vi "Real-Time Main-Final_Local_Digital_V2.vi"() -> ()   [LabVIEW 2024]
uses:
  <instrlib>/niScope/Controls/niScope trigger source digital.ctl
  <vilib>/Platform/TimedLoop/XDataNode/timing_clust.ctl
  <vilib>/Platform/TimedLoop/XDataNode/nitl_modes.ctl
  <vilib>/Platform/TimedLoop/XDataNode/wakeup.ctl
  <instrlib>/niScope/Configure/Trigger/niScope Configure Trigger Digital.vi
  <instrlib>/niScope/Acquire/Fetch/niScope Fetch WDT.vi
  <vilib>/Waveform/WDTOps.llb/WDT Get Waveform Time Array DBL.vi
  <vilib>/platform/TimedLoop/XDataNode/XDataNode.xnode
  <vilib>/Platform/TimedLoop/XDataNode/XDNodeRunTimeDep.lvlib
panel:
  in  "channels":string="0"
  in  "FileName":string
  out "# of Chunks Fetched":i32
  out "# of Points Fetched":i32
  in  "stop":bool
  in  "Fetch:Fetch Relative To":i32(ring)=482 items=["Start"=482, "Trigger"=483, "Pretrigger"=477, "Now"=481, "Read Pointer"=388]
  out "wfm":waveform(dbl)(graph)
  out "Time_shift":dbl
  in  "Resource Name":refnum<k15>="Dev1" caption="Resource Name(s)"
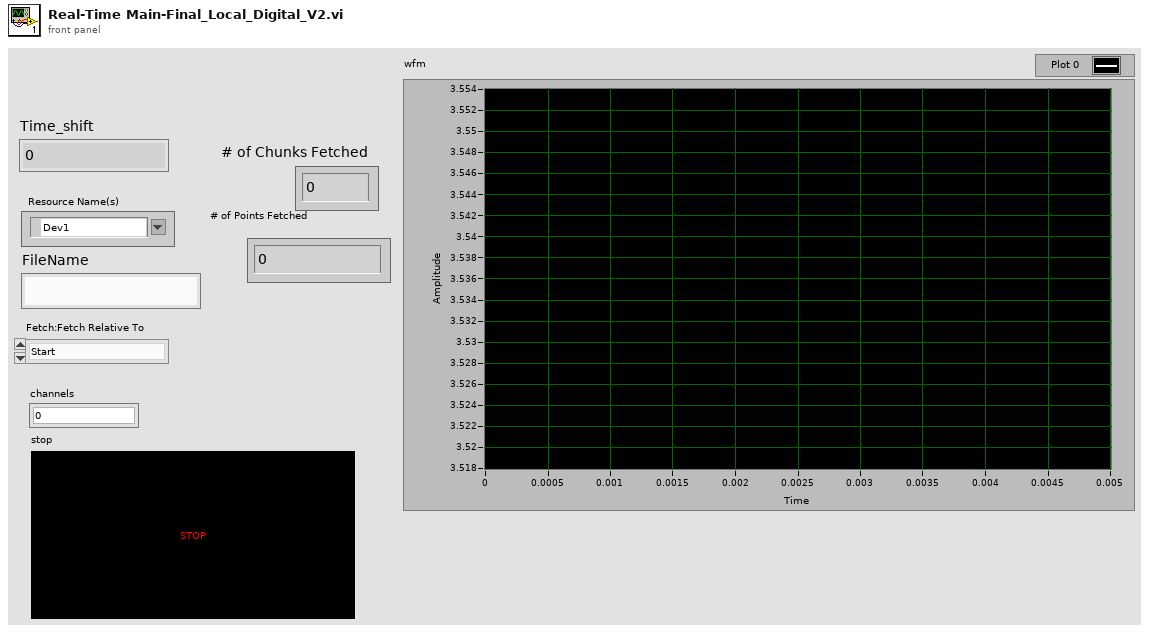
[diagram p1: front panel]
types:
  T1 = typedef "niScope trigger source digital.ctl" = string
  T2 = enum16{"open", "open or create", "create or replace", "create", "open (read-only)"}
  T3 = typedef "XDNodeRunTimeDep.lvlib/timing_clust.ctl" = cluster{"Expected End [f-1]":u64, "Actual End [f-1]":u64, "Finished Late? [f-1]":bool, "Expected End [i-1]":u64, "Actual End [i-1]":u64, "Finished Late? [i-1]":bool, "Expected Start [i]":u64, "Actual Start [i]":u64, "Expected Start [f]":u64, "Actual Start [f]":u64, "Source Name":string, "Structure Name":string, "Period":i64, "Deadline":i64, "Offset":i64, "Start":i64, "Priority":i32, "Timeout":i32, "Mode":T4, "Wakeup Reason":T5, "Error":errorcluster, "Source Type":string, "Secondary Source Type":string, "Global End Time":u64, "Global Start Time":u64, "Frame Duration":u64, "Iteration Duration":u64, "Assigned CPU":i32, "I/O Scan Engine Mode":u32}
  T4 = typedef "XDNodeRunTimeDep.lvlib/nitl_modes.ctl" = enum32{"No Change", "Process missed periods, maintain original phase", "Discard missed periods, maintain original phase", "Process missed periods, ignore original phase", "Discard missed periods, ignore original phase"}
  T5 = typedef "XDNodeRunTimeDep.lvlib/wakeup.ctl" = enum32{"Normal", "Aborted", "Asynchronous wakeup", "Timing source error", "Timed loop error", "Timeout"}
  T6 = cluster{"actualSamples":i32, "absoluteInitialX":dbl, "relativeInitialX":dbl, "xIncrement":dbl, "offset":dbl, "gain":dbl, "reserved1":dbl, "reserved2":dbl}
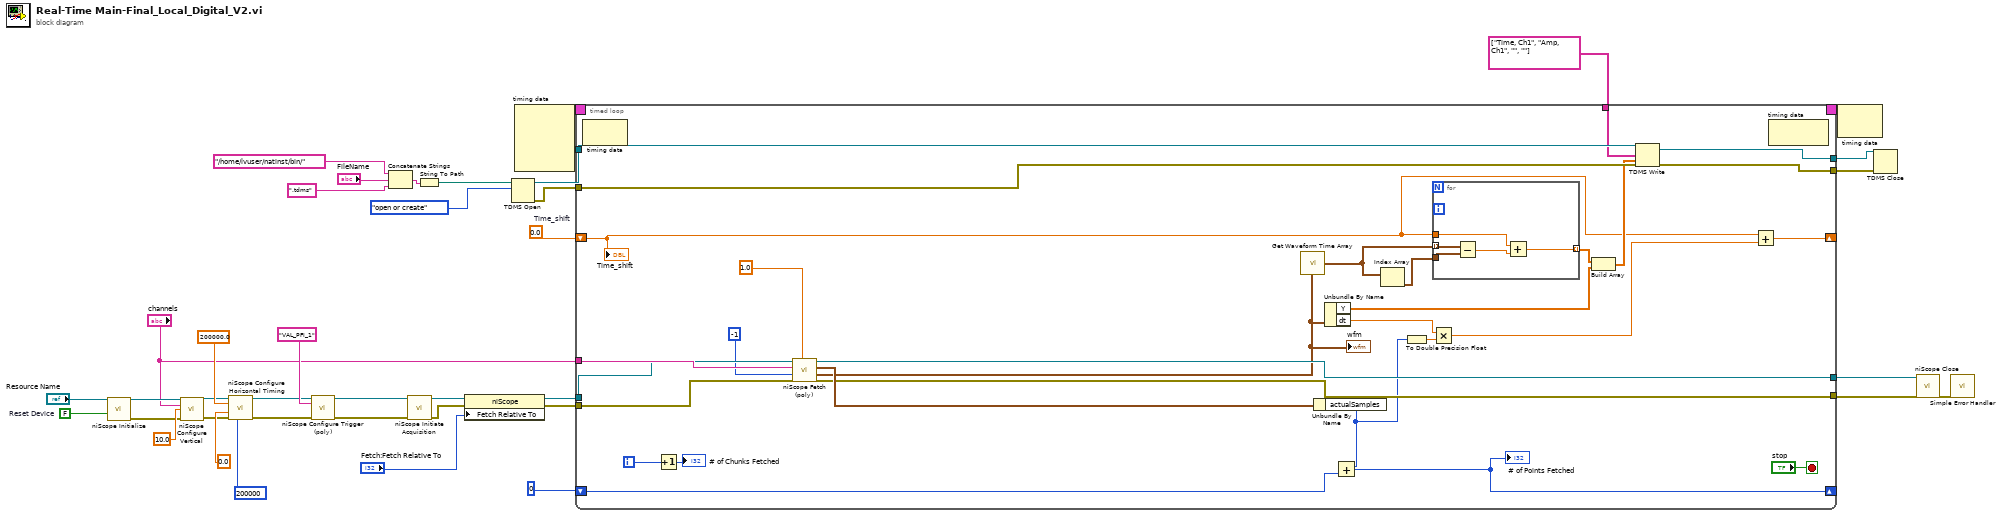
[diagram p0: block diagram]
diagram:
  w25 = 0.0  # Time_shift
  w37 = FALSE  # Reset Device
  n1 = call <instrlib>:"niScope Initialize.vi"("resource name"="Resource Name", "reset device"=w37) -> ("instrument handle"=w14:refnum<k15>, "error out"=w12:errorcluster)  [unwired: 12 in]
  n2 = call <instrlib>:"niScope Configure Vertical.vi"("instrument handle"=w14, "channels"="channels", "vertical range"=10.0, "error in"=w12) -> ("instrument handle out"=w15:refnum<k15>, "error out"=w17:errorcluster)  [unwired: 10 in]
  n3 = call <instrlib>:"niScope Configure Horizontal Timing.vi"("instrument handle"=w15, "min sample rate"=200000.0, "reference position"=0.0, "error in"=w17, "min record length"=200000) -> ("instrument handle out"=w10:refnum<k15>, "error out"=w9:errorcluster)  [unwired: 9 in]
  n4 = call-poly <instrlib>:"niScope Configure Trigger (poly).vi"("instrument handle"=w10, "trigger source"=T1 "VAL_PFI_1", "error in"=w9) -> ("instrument handle out"=w7:refnum<k15>, "error out"=w6:errorcluster)  [unwired: 11 in]
  n5 = Concatenate Strings("/home/lvuser/natinst/bin/" ("string"), "FileName", ".tdms" ("string")) -> (w24:string)
  n6 = call <instrlib>:"niScope Initiate Acquisition.vi"("instrument handle"=w7, "error in"=w6) -> ("instrument handle out"=w4:refnum<k15>, "error out"=w3:errorcluster)  [unwired: 12 in]
  n7 = String To Path(string=w24) -> (path=w22:path)
  n8 = property class="niScope"(reference=w4, error in=w3, "Fetch Relative To"="Fetch:Fetch Relative To") -> (reference out=w2:refnum<k15>, error out=w1:errorcluster)
  n9 = TDMS Open(10:T2."open or create" ("operation (0:open)"), 11:w22) -> (0:w28:errorcluster, 3:w27:refnum<k34>)  [unwired: 5 in]
  n10 = node-c288() -> (w39:T3)  [unwired: 4 in]
  n11 = timed-loop {
    timing: w39 -> [_]
    timing-out: [_] -> w38
    tunnel: [w68] -> w35
    shift-right: [w66] -> _
    shift-left: 0 -> [w67]
    tunnel: [w57] -> w32
    tunnel: w27 -> [w62]
    tunnel: w28 -> [w61]
    tunnel: [w60] -> w30
    tunnel: [w59] -> w29
    tunnel: string[] ["Time, Ch1", "Amp, Ch1", "", ""] ("channel name(s) in (Untitled)") -> [w58]
    shift-right: [w49] -> _
    shift-left: w25 -> [w48]
    tunnel: "channels" -> [w44]
    tunnel: w2 -> [w42]
    tunnel: w1 -> [w40]
    i -> [w65]
    stop <- "stop" stop-if-true
    n12 = node-c288() -> ()  [unwired: 1 in, 1 out]
    n13 = Increment(x=w65) -> (x+1=→"# of Chunks Fetched":i32)
    n14 = call-poly <instrlib>:"niScope Fetch (poly).vi"("timeout"=1.0, "error in"=w40, "numSamples"=-1, "channels"=w44, "instrument handle"=w42) -> ("error out"=w57:errorcluster, "wfm"=w51:waveform(dbl), "wfm info"=w64:T6, "instrument handle out"=w68:refnum<k15>)  [unwired: 3 in]
    "wfm" <- w51
    n15 = call-poly <vilib>:"Get Waveform Time Array.vi"("waveform in"=w51) -> ("X array"=w52:timestamp[])  [unwired: 9 in, 1 out]
    n16 = Unbundle By Name(w64) -> ("actualSamples"=w47:i32)
    n17 = Unbundle By Name(w51) -> ("Y"=w56:dbl[], "dt"=w46:dbl)
    n18 = Add(x=w47, y=w67) -> (x+y=w66:i32)
    "# of Points Fetched" <- w66
    n19 = Index Array(array=w52) -> (element=w53:timestamp)  [unwired: 1 in]
    n20 = To Double Precision Float(number=w47) -> (double precision float=w50:dbl)
    n21 = Multiply(x=w46, y=w50) -> (x*y=w45:dbl)
    n22 = for {
      tunnel: [w72] -> w54 mode=indexing
      tunnel: w53 -> [w74]
      tunnel: w52 -> [w73] mode=indexing
      tunnel: w48 -> [w70]
      n23 = Subtract(x=w73, y=w74) -> (x-y=w71:dbl)
      n24 = Add(x=w70, y=w71) -> (x+y=w72:dbl)
    }
    n25 = Build Array(w54, w56) -> (w55:dbl[][])
    n26 = TDMS Write(0:w62, 7:w58, 9:w55, 11:w61) -> (4:w60:refnum<k34>, 15:w59:errorcluster)  [unwired: 2 in, 2 out]
    n27 = Add(x=w48, y=w45) -> (x+y=w49:dbl)
    n28 = node-c288() -> ()  [unwired: 1 in, 1 out]
    "Time_shift" <- w48
  }
  n29 = node-c288(w38) -> ()  [unwired: 1 out]
  n30 = TDMS Close(8:w29, 11:w30) -> ()  [unwired: 2 out]
  n31 = call <instrlib>:"niScope Close.vi"("instrument handle"=w35, "error in"=w32) -> ("error out"=w33:errorcluster)  [unwired: 13 in]
  n32 = call <vilib>:"Simple Error Handler.vi"("error in (no error)"=w33) -> ()  [unwired: 4 in, 5 out]
